vi "Control System with R and T displays.vi"() -> ()   [LabVIEW 2012]
doc: "Application example"
panel:
  out "CALIBRATION FILE (CH)":string[](array[string])
  in  "CONTROL":u8(ring) items=["ACTIVE", "HOLD"]
  out "CALC SET POINT":sgl format="%^_5e"
  out "RESISTANCE UNIT":string
  out "TEMPERATURE UNIT 2":string
  in  "SET POINT IS GIVEN AS":enum16{"RESISTANCE", "TEMPERATURE"}(ring)
  out "T PAST CAL RANGE":bool
  out "R PAST CAL RANGE":bool
  out "TEMPERATURE UNIT":string
  out "TEMPERATURE (MEAS)":dbl
  in  "HEATER R (OHMS)":dbl=100.0 min=0.0 max=1000.0 step=1.0 format="%#_3f"
  in  "dR/dT":bool
  in  "GIVE SET POINT":dbl min=-1000.0 max=1000.0 format="%^_5e"
  out "HEATER POWER (W)":dbl format="%^_2e"
  out "HEATER CURRENT (A)":dbl format="%^_2e"
  out "HEATER VOLTAGE (V)":dbl format="%^_2e"
  out "% OF AVAILABLE\n       POWER":dbl(knob) scale=0.0..100.0 scale format="%1d"
  out "CONTROL \n   ERROR":dbl(knob) scale=-1.0..1.0 scale format="%.1f"
  out "UPDATING\nDISPLAYS":bool
  in  "NEXT":dbl format="%#_11g"
  in  "INTERVAL (SEC)":T1(ring)
  out "RUNNING":bool
  in  "POWER RANGE":u8(ring) items=["OFF", "1uW", "10uW", "100uW", "1mW", "10mW", "100mW", "1W", ""]
  in  "POWER BIAS":u8(ring) items=["0", "20%", "40%", "60%", "80%", "100%", ""]
  in  "DERIVATOR":u8(ring) items=["0", "1s", "2s", "5s", "10s", "20s", "50s", "100s", ""]
  in  "INTEGRATOR":u8(ring) items=["PD", "2s", "5s", "10s", "20s", "50s", "100s", "200s", "500s", "1000", "LATCHED", "PD", "N/A", "N/A", "N/A", "SHORTED"]
  in  "PROP.  GAIN":u8(ring) items=["5dB", "10dB", "15dB", "20dB", "25dB", "30dB", "35dB", "40dB", "45dB", "50dB", "55dB", "60dB", "N/A", "N/A", "N/A", "SHORTED"]
  in  "stop":bool
  out "RESISTANCE (MEASURED)":sgl format="%^_5e"
  in  "DISPLAY":u8(ring) items=["R", "DR", "ADJ REF", "REFERENCE", "EXC VOLT", "530A HEAT V", "530A HEAT I", "530A SET PT"]
  in  "EXCITATION":u8(ring)=7 items=["NO EXCITATION", "3 uV", "10uV", "30uV", "100uV", "300uV", "1mV", "3mV"]
  in  "RANGE":u8(ring)=3 items=["NO RANGE", "2 Ohms", "20 Ohms", "200 Ohms", "2 kOhms", "20 kOhms", "200 kOhms", "2 MOhms"]
  in  "CHANNEL":u8(ring) items=["CH0", "CH1", "CH2", "CH3", "CH4", "CH5", "CH6", "CH7"]
  in  "INPUT":u8(ring)=2 items=["ZERO", "MEAS", "CAL"]
  out "ADC OVERRANGE":bool
  # "Control System with R and T displays.vi"
  # "AVS-47B"
  # "TS-530A"
  # "OHMS"
  # "OHMS"
  # "SENSOR POLARITY"
  # "Etc....."
  # "This VI is more complicated than the \"Temperature Control System with R display.vi\".   It has the additional features of \n- displaying results as temperature if an R/T calibration file exists.\n- set point can be given as resistance or temperature\n- a \"HOLD\" control setting can be used for measuring other sensors than the control sensor. Hold should be used\n  only for a short time and when the system is at or near to balance.  In hold position, the control is not active but\n  the analog PID integrator maintains the heater power. The system will sooner or later drift away from balance in the \n   HOLD position.\n- readings that are either lower than the first breakpoint resistance or higher than the last breakpoint return\n   temperatures of these breakpoints and set the \"r past cal range\" indicator.\n- set point temperature that is either lower or higher than the lowest or highest breakpoint temperature return\n   resistances of these breakpoints and set the \"t past cal range\" indicator.\n\nThe first lines of the calibration (conversion) file are shown on the left. Nine first rows of these simple text files\ncan be used for customer's and/or sensor manufacturer's purposes. A useful item would be the sensor's location\nin the cryostat.\n\nSee also the descriptions of the  \"Temperature Control System with R display.vi\"."
  # "+"
  # "-"
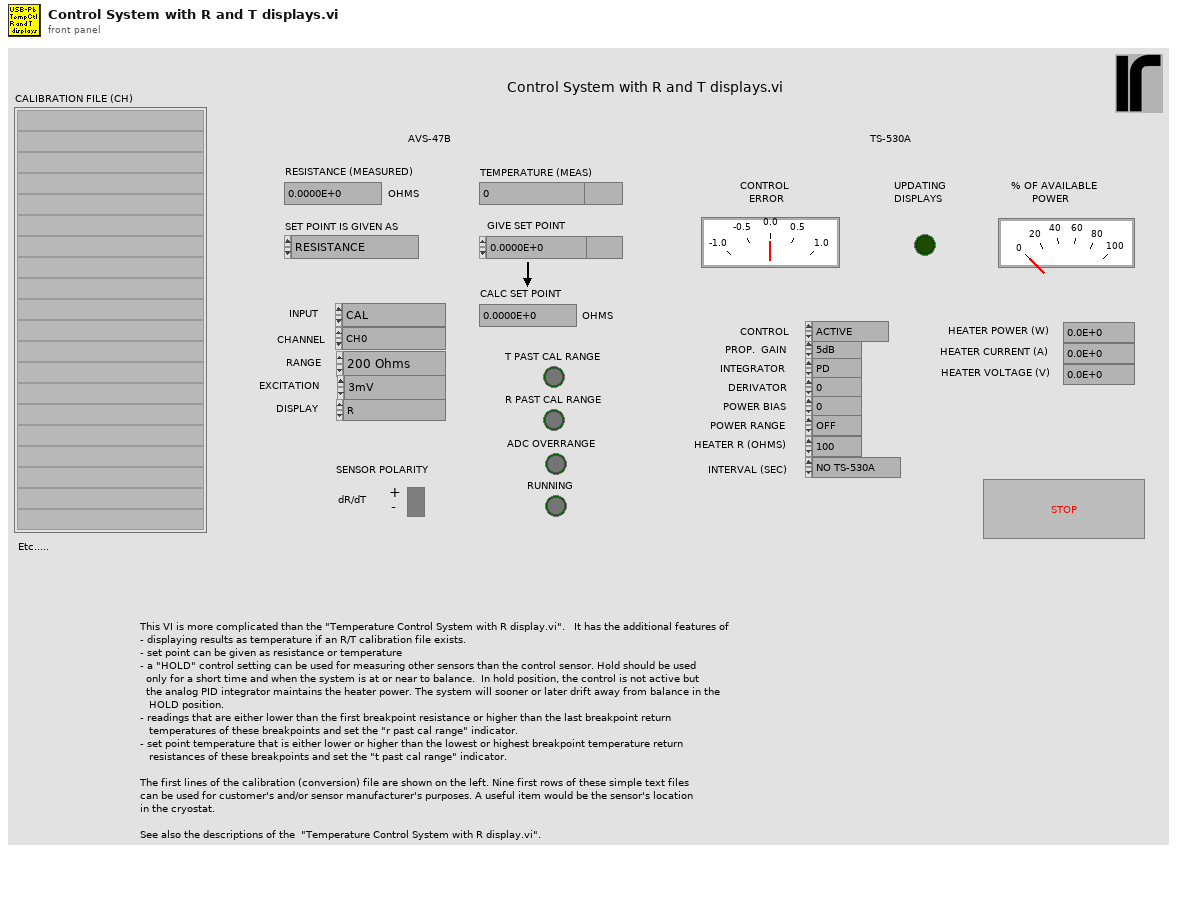
[diagram p1: front panel]
types:
  T1 = enum16{"NO TS-530A", "1", "15", "30", "60", "120", "240"}
  T2 = enum16{"NONE", "READ", "READ AND EDIT", "DEFAULTS"}
  T3 = cluster{"VISA RESOURCE":refnum<visa-resource-name>, "PICOBUS ADDRESS":u8, "DISABLE AL":u8, "REMOTE":u8, "INPUT":u8, "CHANNEL":u8, "RANGE":u8, "EXCITATION":u8, "DISPLAY":u8, "DIGITAL REFERENCE":u16, "SET POINT":dbl, "PROP GAIN":u8, "INTG":u8, "DERIV":u8, "POWER BIAS":u8, "POWER RANGE":u8, "INFO STRING":string, "HEATER RESISTANCE":dbl, "INTERVAL":u8, " SENSOR dR/dT":u8}
  T4 = cluster{"NUMBER OF POINTS":i32, "SIGN OF dT/dR":enum16{"POSITIVE", "NEGATIVE"}, "R/T FORMAT ":enum16{"R", "LOG(R)"}, "TEMPERATURE SCALE":enum16{"KELVINS", "CELSIUS"}, "FILE OK":i32}[]
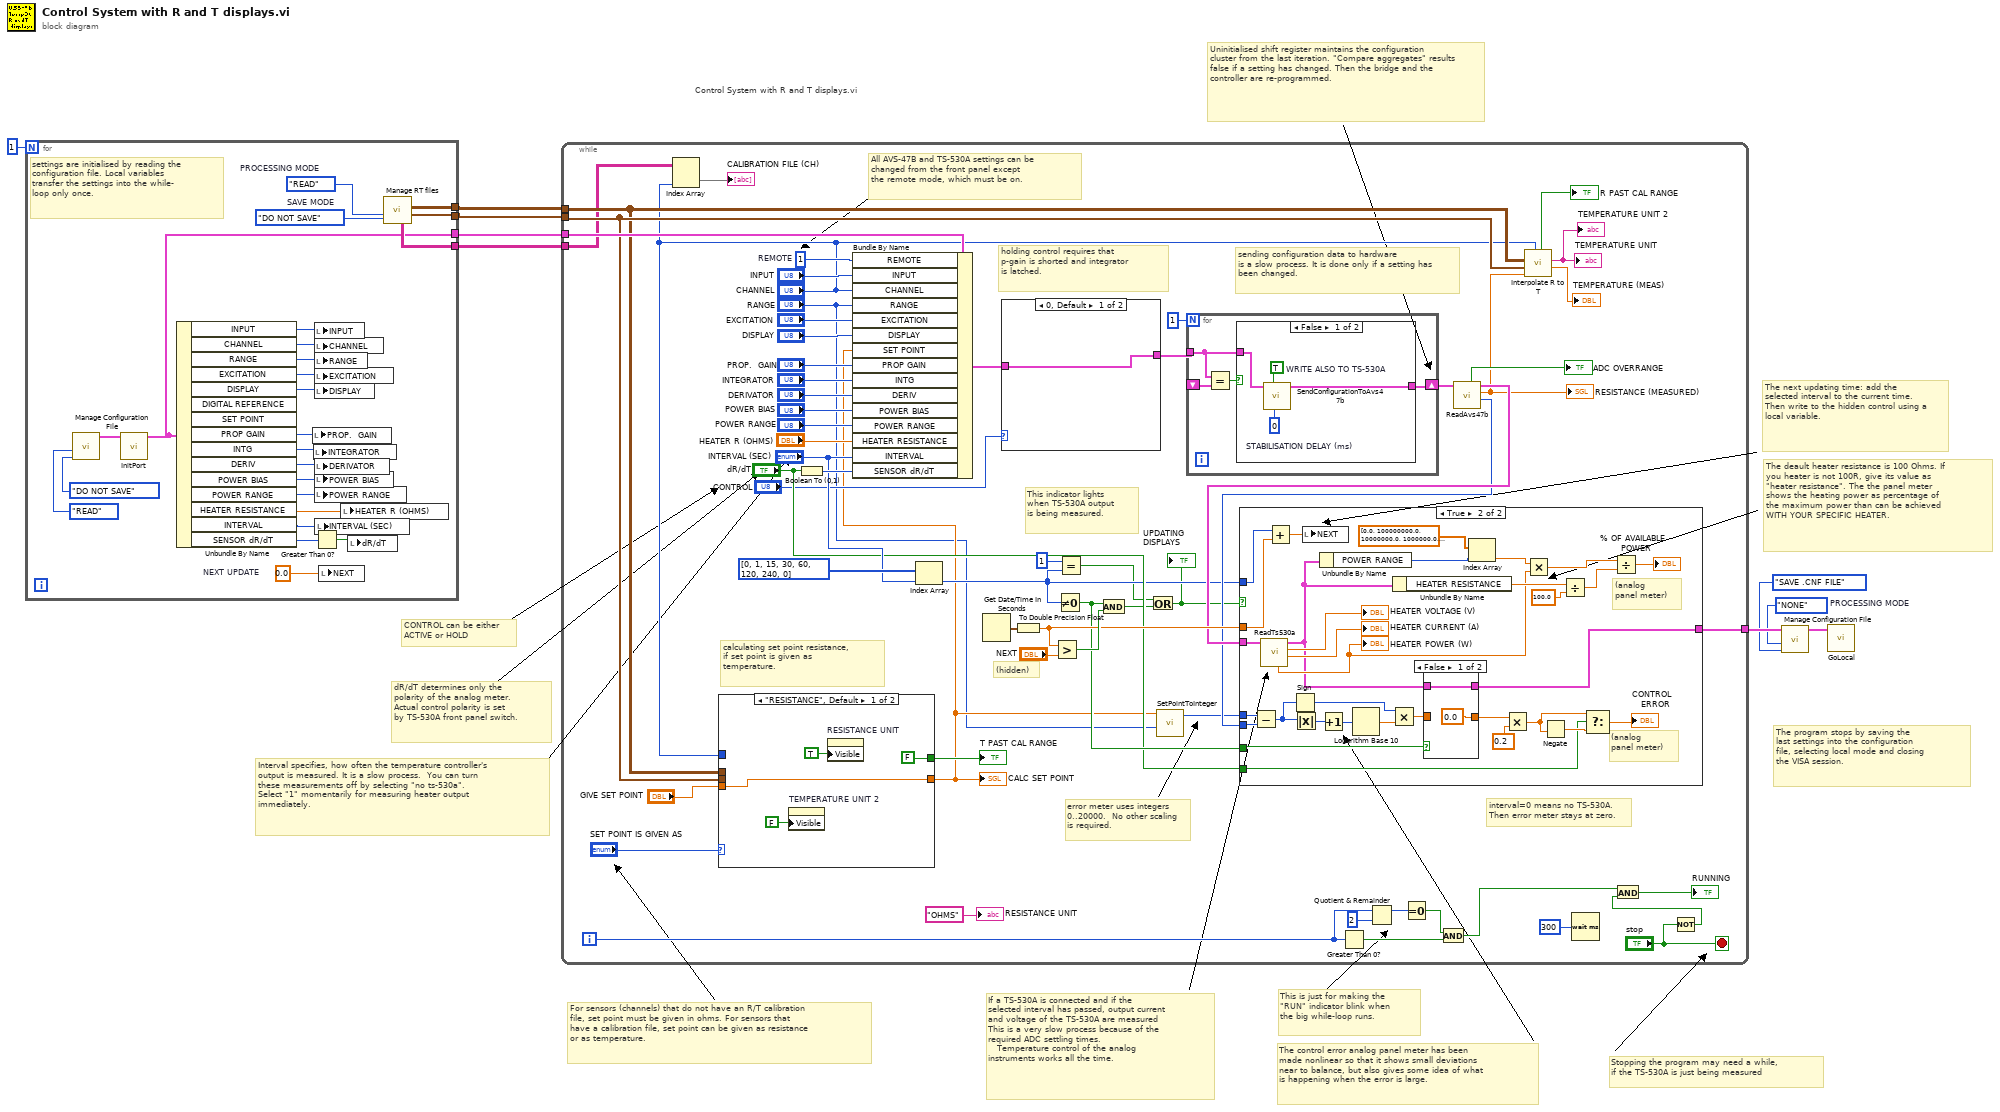
[diagram p0: block diagram]
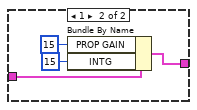
[diagram p2: hidden frame]
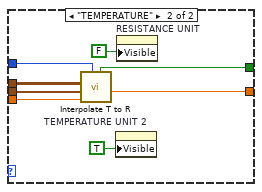
[diagram p3: hidden frame]
diagram:
  w2 = enum16{"NONE", "READ", "CREATE"}."NONE"  # PROCESSING MODE
  # "CONTROL can be either\nACTIVE or HOLD"
  # "The program stops by saving the\nlast settings into the configuration\nfile, selecting local mode and closing \nthe VISA session."
  # "For sensors (channels) that do not have an R/T calibration\nfile, set point must be given in ohms. For sensors that \nhave a calibration file, set point can be given as resistance\nor as temperature."
  # "Uninitialised shift register maintains the configuration\ncluster from the last iteration. \"Compare aggregates\" results false if a setting has changed. Then the bridge and the controller are re-programmed."
  # "The next updating time: add the\nselected interval to the current time. Then write to the hidden control using a local variable."
  # "The deault heater resistance is 100 Ohms. If\nyou heater is not 100R, give its value as \n\"heater resistance\". The the panel meter \nshows the heating power as percentage of\nthe maximum power than can be achieved\nWITH YOUR SPECIFIC HEATER."
  # "Stopping the program may need a while,\nif the TS-530A is just being measured"
  # "The control error analog panel meter has been\nmade nonlinear so that it shows small deviations\nnear to balance, but also gives some idea of what\nis happening when the error is large."
  # "If a TS-530A is connected and if the\nselected interval has passed, output current\nand voltage of the TS-530A are measured\nThis is a very slow process because of the \nrequired ADC settling times.\n   Temperature control of the analog\ninstruments works all the time."
  # "This is just for making the\n\"RUN\" indicator blink when\nthe big while-loop runs."
  # "Interval specifies, how often the temperature controller's\noutput is measured. It is a slow process.  You can turn\nthese measurements off by selecting \"no ts-530a\". \nSelect \"1\" momentarily for measuring heater output\nimmediately."
  # "dR/dT determines only the\npolarity of the analog meter.\nActual control polarity is set\nby TS-530A front panel switch."
  # "Control System with R and T displays.vi"
  n1 = for {
    N: 1 -> [_]
    tunnel: [w12] -> w8
    tunnel: [w18] -> w7
    tunnel: [w17] -> w6
    tunnel: [w16] -> w5
    w10 = enum16{"DO NOT SAVE", "SAVE .CNF FILE"}."DO NOT SAVE"  # SAVE MODE
    w11 = T2."READ"  # PROCESSING MODE
    w23 = 0.0  # NEXT UPDATE
    # "settings are initialised by reading the\nconfiguration file. Local variables\ntransfer the settings into the while-\nloop only once."
    n2 = call "Manage Configuration File.vi"("SAVE MODE"=enum16{"DO NOT SAVE", "SAVE .CNF FILE"}."DO NOT SAVE", "PROCESSING MODE"=enum16{"NONE", "READ", "CREATE"}."READ") -> ("CONFIGURATION CLUSTER OUT"=w13:T3)  [unwired: 9 in]
    n3 = call "InitPort.vi"("CONFIGURATION CLUSTER"=w13) -> ("UNMODIFIED CONFIGURATION CLUSTER"=w12:T3)  [unwired: 6 in, 2 out]
    n4 = Unbundle By Name(w12) -> ("INPUT"=w33:u8, "CHANNEL"=w32:u8, "RANGE"=w31:u8, "EXCITATION"=w30:u8, "DISPLAY"=w29:u8, "PROP GAIN"=w28:u8, "INTG"=w27:u8, "DERIV"=w26:u8, "POWER BIAS"=w25:u8, "POWER RANGE"=w24:u8, "HEATER RESISTANCE"=w19:dbl, "INTERVAL"=w20:u8, "SENSOR dR/dT"=w22:u8)  [unwired: 2 out]
    n5 = local write "PROP.  GAIN"(w28) -> ()
    n6 = local write "INTEGRATOR"(w27) -> ()
    n7 = Greater Than 0?(x=w22) -> (x > 0?=w21:bool)
    n8 = local write "INPUT"(w33) -> ()
    n9 = local write "CHANNEL"(w32) -> ()
    n10 = local write "RANGE"(w31) -> ()
    n11 = local write "EXCITATION"(w30) -> ()
    n12 = local write "DISPLAY"(w29) -> ()
    n13 = local write "DERIVATOR"(w26) -> ()
    n14 = local write "POWER BIAS"(w25) -> ()
    n15 = local write "POWER RANGE"(w24) -> ()
    n16 = local write "INTERVAL (SEC)"(w20) -> ()
    n17 = local write "NEXT"(w23) -> ()
    n18 = local write "HEATER R (OHMS)"(w19) -> ()
    n19 = local write "dR/dT"(w21) -> ()
    n20 = call "Manage RT files.vi"("SAVE MODE"=w10, "PROCESSING MODE"=w11) -> ("FILE INFO"=w17:T4, "R/T BREAKPOINTS"=w18:cluster{dbl, dbl}[][], "COMMENT AREA (9 FIRST ROWS)"=w16:string[][])  [unwired: 5 in, 2 out]
  }
  n21 = while {
    tunnel: [w63] -> w3
    tunnel: w8 -> [w89]
    tunnel: w7 -> [w51]
    tunnel: w6 -> [w52]
    tunnel: w5 -> [w38]
    i -> [w78]
    stop <- "stop" stop-if-true
    w82 = u8 1  # REMOTE
    # "error meter uses integers\n0..20000.  No other scaling\nis required."
    # "interval=0 means no TS-530A.\nThen error meter stays at zero."
    # "calculating set point resistance,\nif set point is given as \ntemperature."
    # "All AVS-47B and TS-530A settings can be\nchanged from the front panel except\nthe remote mode, which must be on."
    # "sending configuration data to hardware\nis a slow process. It is done only if a setting has been changed."
    # "holding control requires that \np-gain is shorted and integrator\nis latched."
    # "This indicator lights\nwhen TS-530A output\nis being measured."
    # "(hidden)"
    n22 = Index Array(array=w38, index (col)="CHANNEL") -> (element=→"CALIBRATION FILE (CH)":string[])  [unwired: 1 in]
    n23 = case shown="\"RESISTANCE\", Default" "SET POINT IS GIVEN AS" {
      tunnel: "GIVE SET POINT" -> [w99 w110]
      tunnel: w52 -> [_ w109]
      tunnel: w51 -> [_ w108]
      tunnel: [w99 w107] -> w35
      tunnel: [FALSE ("T PAST CALIBRATION RANGE") w106] -> w50
      tunnel: "CHANNEL" -> [_ w103]
      frame "RESISTANCE", Default {
        n24 = property on="TEMPERATURE UNIT 2" class="Str"("Visible"=FALSE) -> ()  [unwired: 2 in, 2 out]
        n25 = property on="RESISTANCE UNIT" class="Str"("Visible"=TRUE) -> ()  [unwired: 2 in, 2 out]
      }
      frame "TEMPERATURE" {
        n26 = call "Interpolate T to R.vi"("CHANNEL"=w103, "TEMPERATURE"=w110, "FILE INFO"=w109, "R/T POINTS"=w108) -> ("RESISTANCE (OHMS)"=w107:dbl, "T PAST CALIBRATION RANGE"=w106:bool)  [unwired: 5 in, 1 out]
        n27 = property on="TEMPERATURE UNIT 2" class="Str"("Visible"=TRUE) -> ()  [unwired: 2 in, 2 out]
        n28 = property on="RESISTANCE UNIT" class="Str"("Visible"=FALSE) -> ()  [unwired: 2 in, 2 out]
      }
    }
    "T PAST CAL RANGE" <- w50
    "CALC SET POINT" <- w35
    n29 = Boolean To (0,1)(Boolean="dR/dT") -> (0, 1=w61:i16)
    n30 = Bundle By Name(cluster=w89, "REMOTE"=w82, "INPUT"="INPUT", "CHANNEL"="CHANNEL", "RANGE"="RANGE", "EXCITATION"="EXCITATION", "DISPLAY"="DISPLAY", "SET POINT"=w35, "PROP GAIN"="PROP.  GAIN", "INTG"="INTEGRATOR", "DERIV"="DERIVATOR", "POWER BIAS"="POWER BIAS", "POWER RANGE"="POWER RANGE", "HEATER RESISTANCE"="HEATER R (OHMS)", "INTERVAL"="INTERVAL (SEC)", "SENSOR dR/dT"=w61) -> (w42:T3)
    n31 = Index Array(array=i32[] [0, 1, 15, 30, 60, 120, 240, 0], index="INTERVAL (SEC)") -> (element=w47:i32)
    n32 = Get Date/Time In Seconds() -> (seconds since 1Jan1904=w70:timestamp)
    n33 = case shown="0, Default" "CONTROL" {
      tunnel: w42 -> [w94 w98]
      tunnel: [w94 w95] -> w41
      frame 0, Default {
      }
      frame 1 {
        n34 = Bundle By Name(cluster=w98, "PROP GAIN"=u8 15, "INTG"=u8 15) -> (w95:T3)
      }
    }
    n35 = To Double Precision Float(number=w70) -> (double precision float=w67:dbl)
    n36 = Greater?(x=w67, y="NEXT") -> (0:w68:bool)
    n37 = Not Equal To 0?(x=w47) -> (x != 0?=w65:bool)
    n38 = Equal?(x=1, y=w47) -> (x = y?=w44:bool)
    n39 = And(x=w65, y=w68) -> (x .and. y?=w45:bool)
    n40 = Or(x=w44, y=w45) -> (x .or. y?=w43:bool)
    "UPDATING\nDISPLAYS" <- w43
    n41 = call "SetPointToInteger.vi"("RANGE"="RANGE", "SP OHMS"=w35) -> ("SP INTEGER"=w36:u16)  [unwired: 9 in]
    n42 = for {
      N: 1 -> [_]
      shift-right: [w148] -> w72
      shift-left: _ -> [w151]
      tunnel: w41 -> [w149]
      n43 = Equal?(x=w149, y=w151) -> (x = y?=w150:bool)
      n44 = case shown="False" w150 {
        tunnel: w149 -> [w153 w156]
        tunnel: [w152 w156] -> w148
        frame False {
          w154 = TRUE  # WRITE ALSO TO TS-530A
          w155 = 0  # STABILISATION DELAY (ms)
          n45 = call "SendConfigurationToAvs47b.vi"("STABILISATION DELAY (ms)"=w155, "WRITE ALSO TO TS-530A"=w154, "CONFIGURATION CLUSTER"=w153) -> ("UNMODIFIED CONFIGURATION CLUSTER"=w152:T3)  [unwired: 5 in, 3 out]
        }
        frame True {
        }
      }
    }
    n46 = Greater Than 0?(x=w78) -> (x > 0?=w74:bool)
    n47 = Quotient & Remainder(x=w78, y=2) -> (x-y*floor(x/y)=w76:i32)  [unwired: 1 out]
    n48 = Equal To 0?(x=w76) -> (x = 0?=w75:bool)
    n49 = And(x=w75, y=w74) -> (x .and. y?=w73:bool)
    n50 = call "ReadAvs47b.vi"("CONFIGURATION CLUSTER"=w72) -> ("ADC"=w64:i32, "RESISTANCE (OHMS)"=w57:sgl, "MODIFIED CONFIGURATION CLUSTER"=w66:T3, "ADC OVERRANGE"=→"ADC OVERRANGE":bool)  [unwired: 5 in, 2 out]
    "RESISTANCE (MEASURED)" <- w57
    n51 = case shown="True" w43 {
      tunnel: w47 -> [_ w143]
      tunnel: w67 -> [_ w142]
      tunnel: w66 -> [w111 w140]
      tunnel: w65 -> [_ w131]
      tunnel: w36 -> [_ w130]
      tunnel: w64 -> [_ w129]
      tunnel: "dR/dT" -> [_ w123]
      tunnel: [w111 w112] -> w63
      frame False {
      }
      frame True {
        # "(analog\npanel meter)"
        # "(analog\npanel meter)"
        n52 = Subtract(x=w130, y=w129) -> (x-y=w138:i32)
        n53 = call "ReadTs530a.vi"("CONFIGURATION CLUSTER"=w140) -> ("HEATER CURRENT"=→"HEATER CURRENT (A)":dbl, "HEATER VOLTAGE"=→"HEATER VOLTAGE (V)":dbl, "UNMODIFIED CONFIGURATION CLUSTER"=w113:T3, "HEATER POWER"=w114:dbl)  [unwired: 6 in, 1 out]
        "HEATER POWER (W)" <- w114
        n54 = Add(x=w143, y=w142) -> (x+y=w141:dbl)
        n55 = Sign(1:w138) -> (0:w137:i32)
        n56 = Absolute Value(x=w138) -> (abs(x)=w135:i32)
        n57 = local write "NEXT"(w141) -> ()
        n58 = Unbundle By Name(w113) -> ("POWER RANGE"=w121:u8)
        n59 = Increment(x=w135) -> (x+1=w134:i32)
        n60 = Logarithm Base 10(1:w134) -> (0:w136:dbl)
        n61 = Multiply(x=w137, y=w136) -> (x*y=w133:dbl)
        n62 = Unbundle By Name(w113) -> ("HEATER RESISTANCE"=w115:dbl)
        n63 = case shown="False" w131 {
          tunnel: w133 -> [_ w147]
          tunnel: [0.0 w147] -> w132
          tunnel: w113 -> [w144 w146]
          tunnel: [w144 w146] -> w112
          frame False {
          }
          frame True {
          }
        }
        n64 = Index Array(array=dbl[] [0.0, 100000000.0, 10000000.0, 1000000.0, 100000.0, 10000.0, 1000.0, 100.0], index=w121) -> (element=w120:dbl)
        n65 = Multiply(x=w132, y=0.2) -> (x*y=w125:dbl)
        n66 = Multiply(x=w120, y=w114) -> (x*y=w117:dbl)
        n67 = Negate(x=w125) -> (-x=w124:dbl)
        n68 = Divide(x=w115, y=100.0) -> (x/y=w118:dbl)
        n69 = Select(t=w125, s=w123, f=w124) -> (s? t:f=→"CONTROL \n   ERROR":dbl)
        n70 = Divide(x=w117, y=w118) -> (x/y=→"% OF AVAILABLE\n       POWER":dbl)
      }
    }
    n71 = call "Interpolate R to T.vi"("CHANNEL"="CHANNEL", "RESISTANCE (OHMS)"=w57, "FILE INFO"=w52, "R/T POINTS"=w51) -> ("TEMPERATURE"=→"TEMPERATURE (MEAS)":dbl, "TEMPERATURE UNIT"=→"TEMPERATURE UNIT" →"TEMPERATURE UNIT 2":string, "R PAST CALIBRATION RANGE"=→"R PAST CAL RANGE":bool)  [unwired: 4 in, 1 out]
    n72 = Wait (ms)(milliseconds to wait=u32 300) -> ()  [unwired: 1 out]
    n73 = Not(x="stop") -> (.not. x?=w79:bool)
    n74 = And(x=w73, y=w79) -> (x .and. y?=→"RUNNING":bool)
    "RESISTANCE UNIT" <- "OHMS" ("RESISTANCE UNIT")
  }
  n75 = call "Manage Configuration File.vi"("SAVE MODE"=enum16{"DO NOT SAVE", "SAVE .CNF FILE"}."SAVE .CNF FILE", "PROCESSING MODE"=w2, "CONFIGURATION CLUSTER"=w3) -> ("CONFIGURATION CLUSTER OUT"=w4:T3)  [unwired: 8 in]
  n76 = call "GoLocal.vi"("CONFIGURATION CLUSTER"=w4) -> ()  [unwired: 10 in, 1 out]
